vi "Validate Configuration (Framework).vi"(8 "error in (no error)":errorcluster, 11 "framework configuration in":T1) -> (0 "error out":errorcluster, 3 "framework configuration out":T1)   [LabVIEW 2017, in "DSF Core.lvlib"]
uses:
  DSF Core.lvlib
  Controls/DSF Timing Info.ctl
  Controls/DSF Settings Info.ctl
  Controls/DSF Engine Plugin Thread Configuration.ctl
  Controls/DSF Direction.ctl
  Controls/DSF Byte Order.ctl
  Controls/DSF Data Type.ctl
  Controls/DSF Channel Buffer Descriptor.ctl
  Controls/DSF Engine Channel Configuration.ctl
  Controls/DSF Engine Transfer Configuration.ctl
  Controls/DSF Engine Transfer Group Configuration.ctl
  Controls/DSF Engine Plugin Configuration.ctl
  Controls/DSF Engine Framework Configuration.ctl
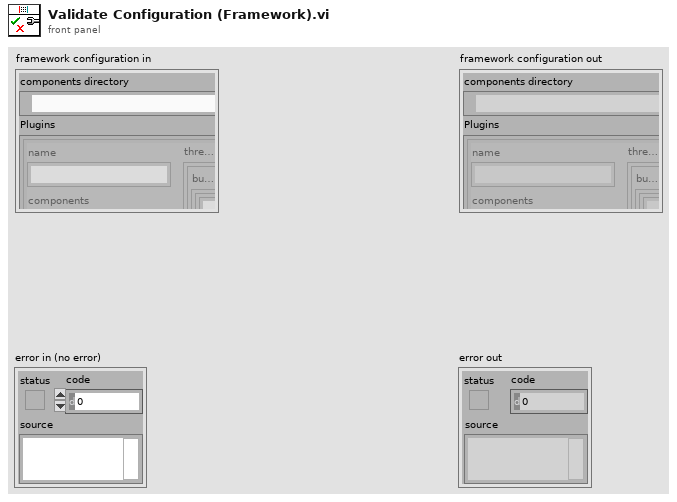
[diagram p1: front panel]
types:
  T1 = typedef "DSF Core.lvlib/DSF Engine Framework Configuration.ctl" = cluster{"components directory":path, "Plugins":T2[]}
  T2 = typedef "DSF Core.lvlib/DSF Engine Plugin Configuration.ctl" = cluster{"name":string, "components":string[], "cycle timing":T3, "threads":T4[], "Transfer Groups":T6[], "settings":T5}
  T3 = typedef "DSF Core.lvlib/DSF Timing Info.ctl" = cluster{"priority":u64, "decimation":u64, "offset":u64}
  T4 = typedef "DSF Core.lvlib/DSF Engine Plugin Thread Configuration.ctl" = cluster{"buffer converter settings":T5, "transceiver settings":T5, "processor":i32}
  T5 = typedef "DSF Core.lvlib/DSF Settings Info.ctl" = cluster{"key":string, "value":string}[]
  T6 = typedef "DSF Core.lvlib/DSF Engine Transfer Group Configuration.ctl" = cluster{"name":string, "direction":T7, "cycle timing":T3, "thread":i32, "settings":T5, "Transfers":T8[]}
  T7 = typedef "DSF Core.lvlib/DSF Direction.ctl" = enum8{"Tx", "Rx"}
  T8 = typedef "DSF Core.lvlib/DSF Engine Transfer Configuration.ctl" = cluster{"name":string, "byte order":T9, "channel blocks":T10[], "settings":T5}
  T9 = typedef "DSF Core.lvlib/DSF Byte Order.ctl" = enum8{"big-endian", "little-endian"}
  T10 = typedef "DSF Core.lvlib/DSF Engine Channel Configuration.ctl" = cluster{"engine descriptor":T11, "string descriptor":T11, "count":u64, "name":string}
  T11 = typedef "DSF Core.lvlib/DSF Channel Buffer Descriptor.ctl" = cluster{"buffer offset":u64, "data type":T12}
  T12 = typedef "DSF Core.lvlib/DSF Data Type.ctl" = enum8{"Bool", "SGL", "DBL", "I8", "I16", "I32", "I64", "U8", "U16", "U32", "U64"}
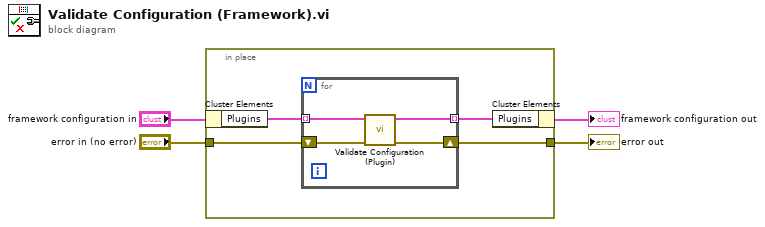
[diagram p0: block diagram]
diagram:
  n1 = in-place {
    in-place-border: "error in (no error)" -> [w6]
    in-place-border: [w5] -> w1
    n2 = in-place-cluster #1("framework configuration in") -> ("Plugins"=w8:T2[])
    n3 = for {
      tunnel: w8 -> [w12] mode=indexing
      tunnel: [w11] -> w7 mode=indexing
      shift-right: [w10] -> w5
      shift-left: w6 -> [w9]
      n4 = call "Validate Configuration (Plugin).vi"("error in (no error)"=w9, "plugin configuration in"=w12) -> ("error out"=w10:errorcluster, "plugin configuration out"=w11:T2)  [unwired: 8 in]
    }
    n5 = in-place-cluster #1("Plugins"=w7) -> (→"framework configuration out":T1)
  }
  "error out" <- w1
